vi "Mock Launch Helper Loop Throwing Error.vi"(8 "error in (no error)":errorcluster, 10 "Error message":errorcluster, 11 "Mock Process in":refnum<class "Mock Process.lvclass">) -> (0 "error out":errorcluster, 3 "Mock Process out":refnum<class "Mock Process.lvclass">)   [LabVIEW 2020, in "Mock Process.lvclass"]
uses:
  Mock Process.lvclass
  C:/Users/anton/Documents/GitHub/Triarc/source/Framework/Helper Loop/Helper Loop.lvclass
  Framework/Helper Loop/Helper Loop.lvclass
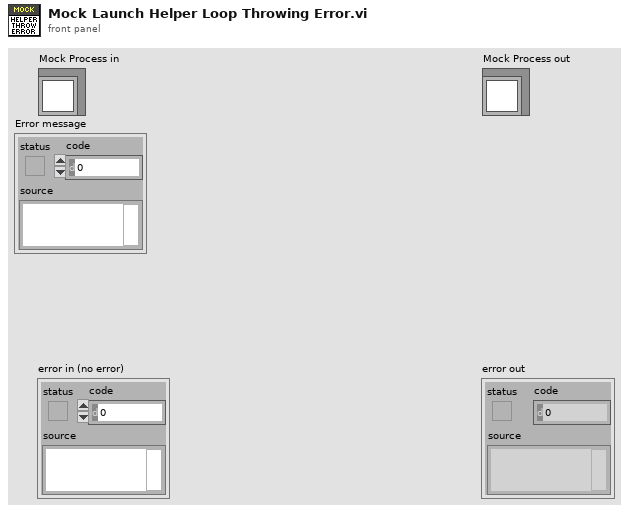
[diagram p1: front panel]
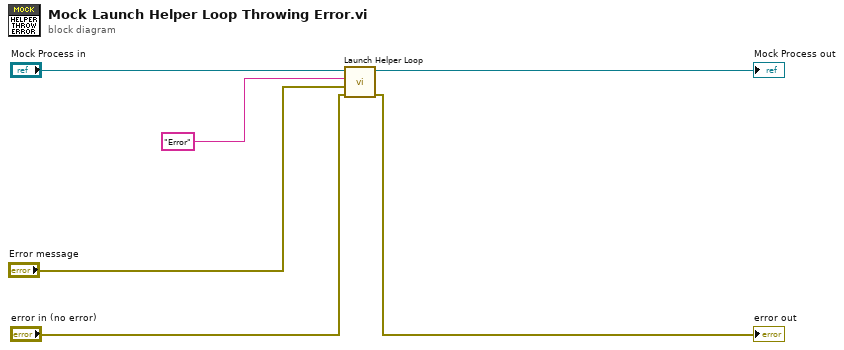
[diagram p0: block diagram]
diagram:
  n1 = call "Launch Helper Loop.vi"("error in (no error)"="error in (no error)", "Message Data"="Error message", "Message"="Error", "Helper Loop In"="Mock Process in") -> ("error out"=→"error out":errorcluster, "Helper Loop Out"=→"Mock Process out":refnum<class "Mock Process.lvclass">)  [unwired: 6 in]
